vi "UTF-8 to Text.vi"(8 "error in":errorcluster, 11 "utf-8 text":string) -> (0 "error out":errorcluster, 3 "text":string)   [LabVIEW 2014, in "SQLite3LV.lvlib"]
uses:
  SQLite3LV.lvlib
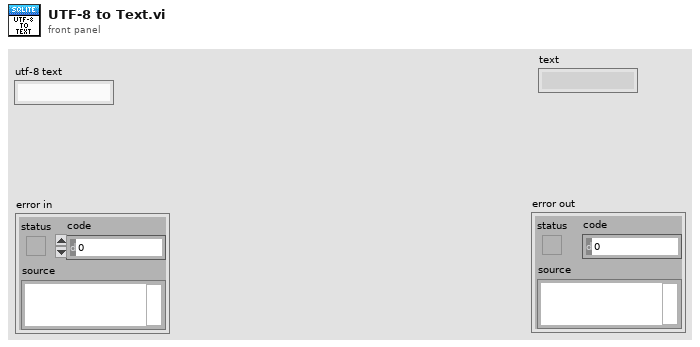
[diagram p1: front panel]
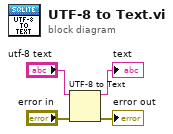
[diagram p0: block diagram]
diagram:
  n1 = UTF-8 to Text(8:"error in", 11:"utf-8 text") -> (0:→"error out":errorcluster, 3:→"text":string)  [unwired: 1 in]
